vi "Unregister.vi"(8 "Error In":errorcluster, 9 "Registrant Enq":refnum<class "Message Enqueuer.lvclass">, 11 "Controller Actor In":refnum<class "Controller Actor.lvclass">) -> (0 "Error Out":errorcluster, 3 "Controller Actor Out":refnum<class "Controller Actor.lvclass">)   [LabVIEW 2017, in "Event Actors.lvlib" / "Controller Actor.lvclass"]
doc: "This method unregisters a specific Actors Enqueuer from all Events he is listening to from this Event Source Actor."
uses:
  Controller Actor.lvclass
  <vilib>/ActorFramework/Message Enqueuer/Message Enqueuer.lvclass
  Controller Actor.lvclass/Controller Actor.ctl
  <resource>/AFDebug/Generate Trace.vi
  <resource>/AFDebug/TDM Registry.vi
  <resource>/AFDebug/Localized Strings.vi
  <resource>/AFDebug/Actor Registry.vi
  <resource>/AFDebug/Get Clone Name.vi
  <resource>/AFDebug/AF Debug.lvlib
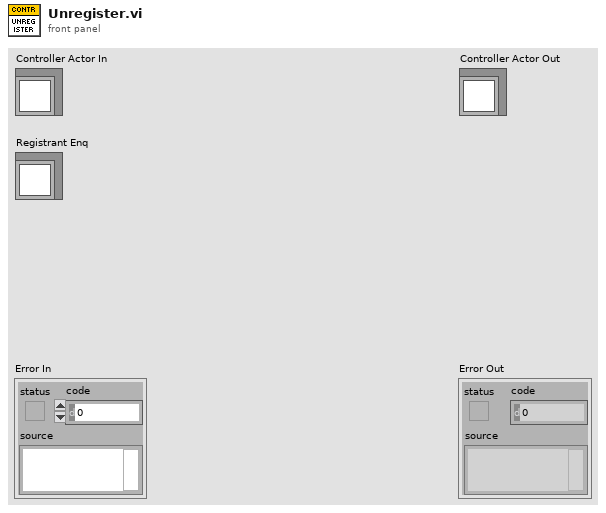
[diagram p1: front panel]
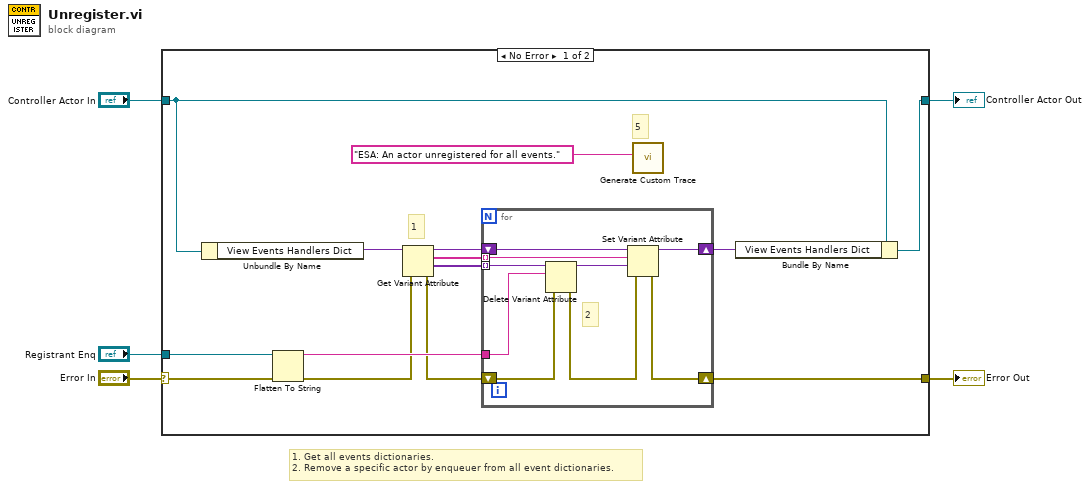
[diagram p0: block diagram]
diagram:
  # "1. Get all events dictionaries.\n2. Remove a specific actor by enqueuer from all event dictionaries."
  n1 = case shown="No Error" "Error In" {
    selector: "Error In" -> [w16 w30]
    tunnel: "Registrant Enq" -> [w19 _]
    tunnel: [w17 w30] -> w4
    tunnel: "Controller Actor In" -> [w9 w29]
    tunnel: [w8 w29] -> w1
    frame No Error {
      # "5"
      # "1"
      n2 = Unbundle By Name(w9) -> ("View Events Handlers Dict"=w15:variant)
      n3 = Flatten To String(anything=w19, error in (no error)=w16) -> (data string=w18:string, error out=w14:errorcluster)  [unwired: 2 in, 1 out]
      n4 = Get Variant Attribute(Variant=w15, error in=w14) -> (duplicate Variant=w10:variant, names=w11:string[], values=w13:variant[], error out=w12:errorcluster)  [unwired: 2 in]
      n5 = for {
        tunnel: w13 -> [w28] mode=indexing
        tunnel: w18 -> [w27]
        shift-right: [w20] -> w17
        shift-left: w12 -> [w26]
        tunnel: w11 -> [w24] mode=indexing
        shift-right: [w22] -> w7
        shift-left: w10 -> [w23]
        # "2"
        n6 = Delete Variant Attribute(4:w26, 6:w27, 7:w28) -> (0:w21:errorcluster, 3:w25:variant)  [unwired: 1 out]
        n7 = Set Variant Attribute(Variant=w23, name=w24, value=w25, error in=w21) -> (Variant out=w22:variant, error out=w20:errorcluster)  [unwired: 1 out]
      }
      n8 = call <resource>:"Generate Custom Trace.vi"("Custom Action"="ESA: An actor unregistered for all events.") -> ()  [unwired: 11 in]
      n9 = Bundle By Name(cluster=w9, "View Events Handlers Dict"=w7) -> (w8:refnum<class "Controller Actor.lvclass">)
    }
    frame Error {
    }
  }
  "Error Out" <- w4
  "Controller Actor Out" <- w1
